vi "Launch.vi"(7 "Common Config":T1={"Launch Timeout [ms]"=-1, "Wait For Launch Completed"=FALSE, "Front Panel State"=enum."Standard", "Close FP On Shutdown"=TRUE, "Response Channel"=refnum, "Sub Panel"=refnum}, 8 "error in (no error)":errorcluster, 10 "Maximum Number Of Errors":i32) -> (0 "error out":errorcluster, 3 "Launch Time":timestamp)   [LabVIEW 2021, in "Error Handler Actor.lvclass"]
doc: "<b>Response</b> channel is used by this actor to return infomation back to the parent. Typically this input is the Request channel of the parent actor."
uses:
  Error Handler Actor.lvclass
  Error Handler Actor.lvclass/Error Handler Actor.ctl
  C:/dev/LabVIEW/LabMelee/Source/Re-use Libraries/Minimal Actor Framework/Actors/Base Actor/Actor/Actor.lvclass
  C:/dev/LabVIEW/LabMelee/Source/Application Specific/Actors/Error Handler/Actor/Error Handler Actor.lvclass
  API/Error Handler Actor API.lvclass
  C:/dev/LabVIEW/LabMelee/Source/Re-use Libraries/Minimal Actor Framework/Actors/Base Actor/API/Actor API.lvclass
  C:/dev/LabVIEW/LabMelee/Source/Application Specific/Actors/Error Handler/API/Error Handler Actor API.lvclass
  Re-use Libraries/Minimal Actor Framework/Actors/Base Actor/API/Actor API.lvclass
  Re-use Libraries/Minimal Actor Framework/Actors/Base Actor/Actor/Actor.lvclass
  Process.vi
  Globals.vi
  Re-use Libraries/Minimal Actor Framework/Messaging/Messenger/Messenger.lvclass
  Re-use Libraries/Minimal Actor Framework/Actors/Base Actor/Actor/Front Panel State.ctl
  Re-use Libraries/Minimal Actor Framework/Actors/Base Actor/Actor/Common Config.ctl
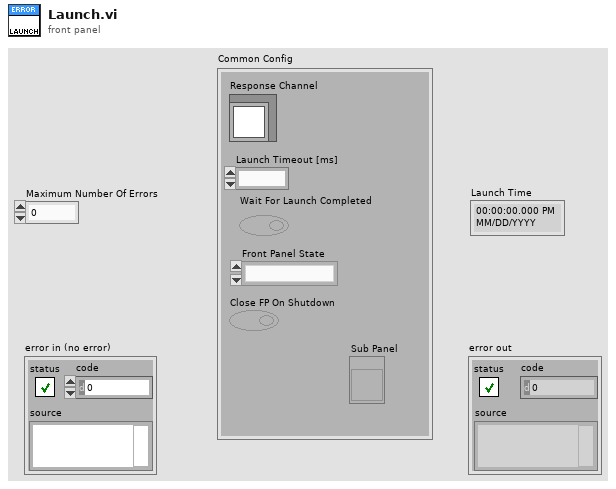
[diagram p1: front panel]
types:
  T1 = typedef "Actor.lvclass/Common Config.ctl" = cluster{"Launch Timeout [ms]":i32, "Wait For Launch Completed":bool, "Front Panel State":T2, "Close FP On Shutdown":bool, "Response Channel":refnum<class "Messenger.lvclass">, "Sub Panel":refnum<vi>}
  T2 = typedef "Actor.lvclass/Front Panel State.ctl" = enum32{"Invalid", "Standard", "Closed", "Hidden", "Minimized", "Maximized"}
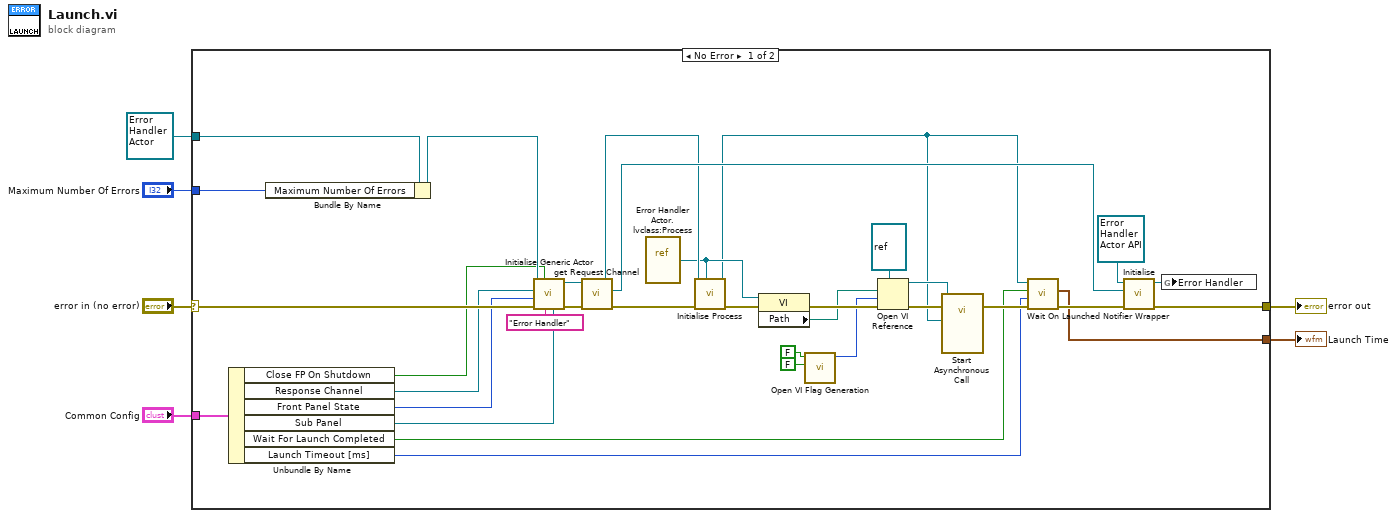
[diagram p0: block diagram]
diagram:
  n1 = case shown="No Error" "error in (no error)" {
    selector: "error in (no error)" -> [w36 w40]
    tunnel: [w35 w40] -> w6
    tunnel: refnum<class "Error Handler Actor.lvclass"> refnum ("Worker Test 1.lvclass") -> [w34 _]
    tunnel: "Maximum Number Of Errors" -> [w32 _]
    tunnel: [w30 _] -> w2
    tunnel: "Common Config" -> [w13 _]
    frame No Error {
      n2 = Unbundle By Name(w13) -> ("Close FP On Shutdown"=w12:bool, "Response Channel"=w11:refnum<class "Messenger.lvclass">, "Front Panel State"=w10:T2, "Sub Panel"=w9:refnum<vi>, "Wait For Launch Completed"=w8:bool, "Launch Timeout [ms]"=w7:i32)
      n3 = Bundle By Name(cluster=w34, "Maximum Number Of Errors"=w32) -> (w33:refnum<class "Error Handler Actor.lvclass">)
      n4 = call-dynamic "Initialise Generic Actor.vi"("Sub Panel"=w9, "Name"="Error Handler", "Close FP On Shutdown (T)"=w12, "Front Panel State"=w10, "Response Channel"=w11, "Actor in"=w33) -> ("Actor out"=w37:refnum<class "Error Handler Actor.lvclass">)  [unwired: 4 in, 1 out]
      n5 = call "get Request Channel.vi"("error in (no error)"=w36, "Actor in"=w37) -> ("error out"=w19:errorcluster, "Request Channel"=w39:refnum<class "Messenger.lvclass">, "Actor out"=w17:refnum<class "Error Handler Actor.lvclass">)  [unwired: 7 in]
      n6 = vi-ref "Error Handler Actor.lvclass:Process.vi"() -> (w16:refnum<vi>)
      n7 = call-dynamic "Initialise Process.vi"("Process"=w16, "error in (no error)"=w19, "Actor in"=w17) -> ("error out"=w28:errorcluster, "Actor out"=w15:refnum<class "Error Handler Actor.lvclass">)  [unwired: 7 in]
      n8 = property class="VI"(reference=w16, error in=w28) -> (error out=w27:errorcluster, "Path"=w20:path)  [unwired: 1 out]
      n9 = call "Open VI Flag Generation.vi"("Call And Collect (F)"=FALSE, "Re-entrant (F)"=FALSE) -> ("Flags"=w26:i32)  [unwired: 9 in]
      n10 = Open VI Reference(type specifier VI Refnum (for type only)=refnum<vi> refnum, vi path=w20, options=w26, error in (no error)=w27) -> (vi reference=w22:refnum<vi>, error out=w21:errorcluster)  [unwired: 2 in]
      n11 = call-by-ref "Start Asynchronous Call"(reference=w22, error in=w21, "Actor"=w15) -> (error out=w18:errorcluster)  [unwired: 11 in, 1 out]
      n12 = call-dynamic "Wait On Launched Notifier Wrapper.vi"("error in (no error)"=w18, "Launch Timeout [ms]"=w7, "Wait For Launch Completed"=w8, "Actor in"=w15) -> ("error out"=w31:errorcluster, "Launch Time"=w30:timestamp)  [unwired: 5 in, 1 out]
      n13 = call "Initialise.vi"("error in (no error)"=w31, "Request Channel"=w39, "Actor API in"=refnum<class "Error Handler Actor API.lvclass"> refnum ("Actor API")) -> ("error out"=w35:errorcluster, "Actor API out"=w14:refnum<class "Error Handler Actor API.lvclass">)  [unwired: 7 in]
      n14 = global write "Globals.vi" "Error Handler"(w14) -> ()
    }
    frame Error {
    }
  }
  "error out" <- w6
  "Launch Time" <- w2
